vi "Create Map from Identifiers to Indexes.vi"(11 "RT hardware channel data":T2[](array[typedef]) {"labels settings for RT"."Label Timestamp Channel Data Reference" format="%.0x"; "labels settings for RT"."Word Initial Raw Value" format="%032.0f"; "labels settings for RT"."Label Disable/Trigger Channel Reference" format="%.0x"; "labels settings for RT"."parameter driver data"."Tx parameter refs" format="%.0x"; "labels settings for RT"."SDI" format="%02b"; "labels settings for RT"."label" format="%.0o"}) -> (3 "map from identifiers to indexes":T1)   [LabVIEW 2021, in "Ballard ARINC 429 Engine.lvlib" / "Custom Device.lvlib"]
uses:
  Custom Device.lvlib
  Shared/Map of Identifiers to Indexes.ctl
  Shared/Label.ctl
  <vilib>/NI/NI VeriStand Encoding and Decoding/Encoding.ctl
  <vilib>/NI/NI VeriStand Encoding and Decoding/Encoding and Decoding.lvlib
  Shared/Parameter Definition.ctl
  <vilib>/NI VeriStand/Custom Device API/Data Reference.ctl
  <vilib>/NI VeriStand/Custom Device API/Custom Device API.lvlib
  <vilib>/NI VeriStand/Custom Device API/Custom Device Item Ref.ctl
  Shared/RT Parameters.ctl
  Shared/Transfer Type.ctl
  Shared/RT Label Settings.ctl
  Shared/RT Hardware Channel Settings.ctl
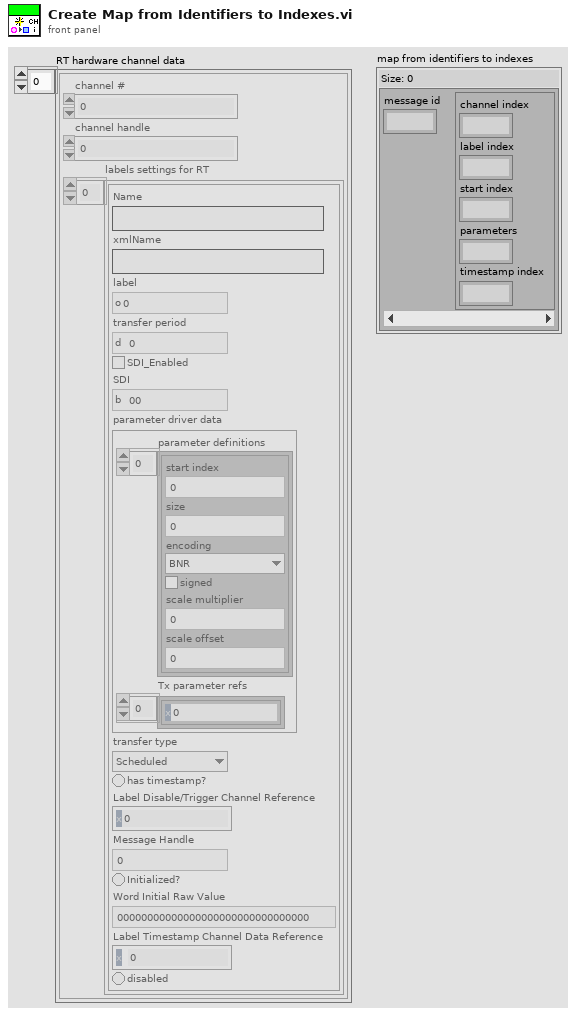
[diagram p1: front panel]
types:
  T1 = typedef "Map of Identifiers to Indexes.ctl" = map{u32, cluster{"channel index":i32, "label index":i32, "start index":i32, "parameters":i32, "timestamp index":i32}}
  T2 = typedef "RT Hardware Channel Settings.ctl" = cluster{"channel #":u16, "channel handle":u64, "labels settings for RT":T3[]}
  T3 = typedef "RT Label Settings.ctl" = cluster{"Name":string, "xmlName":string, "label":T4, "transfer period":u32, "SDI_Enabled":bool, "SDI":u8, "parameter driver data":T5, "transfer type":T9, "has timestamp?":bool, "Label Disable/Trigger Channel Reference":T8, "Message Handle":u64, "Initialized?":bool, "Word Initial Raw Value":u32, "Label Timestamp Channel Data Reference":T10, "disabled":bool}
  T4 = typedef "Label.ctl" = u8
  T5 = typedef "RT Parameters.ctl" = cluster{"parameter definitions":T6[], "Tx parameter refs":T8[]}
  T6 = typedef "Parameter Definition.ctl" = cluster{"start index":i32, "size":i32, "encoding":T7, "signed":bool, "scale multiplier":dbl, "scale offset":dbl}
  T7 = typedef "Encoding and Decoding.lvlib/Encoding.ctl" = enum16{"BNR", "BCD", "Discrete"}
  T8 = typedef "Custom Device API.lvlib/Custom Device Item Ref.ctl" = u64
  T9 = typedef "Transfer Type.ctl" = enum16{"Scheduled", "Acyclic", "Block", "Strobe"}
  T10 = typedef "Custom Device API.lvlib/Data Reference.ctl" = i32
  T11 = cluster{"channel index":i32, "label index":i32, "start index":i32, "parameters":i32, "timestamp index":i32}
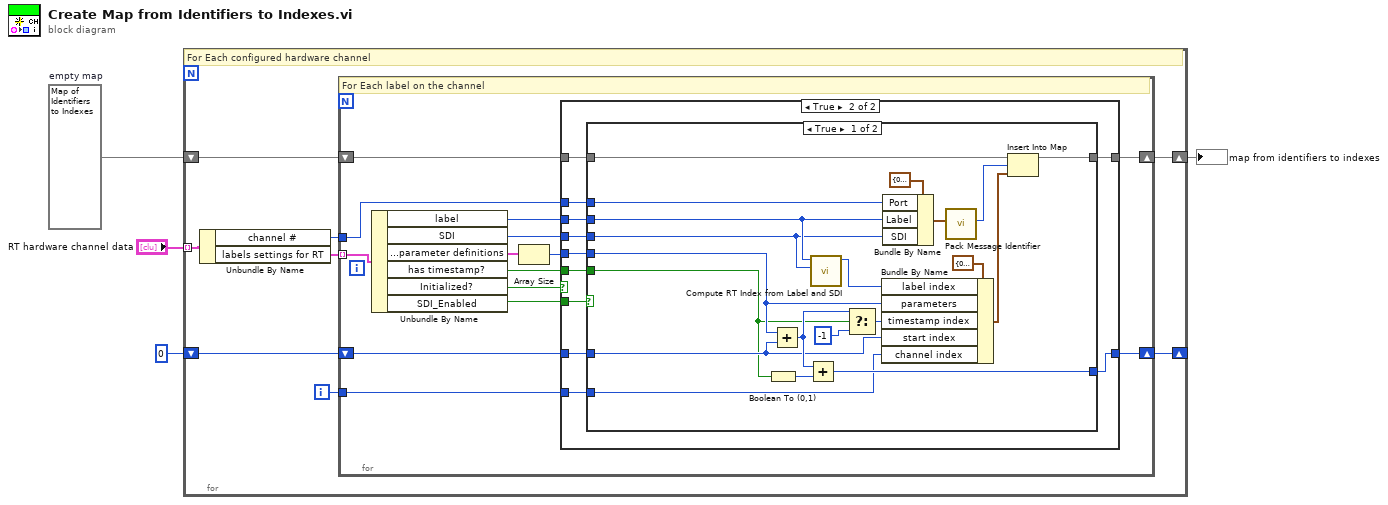
[diagram p0: block diagram]
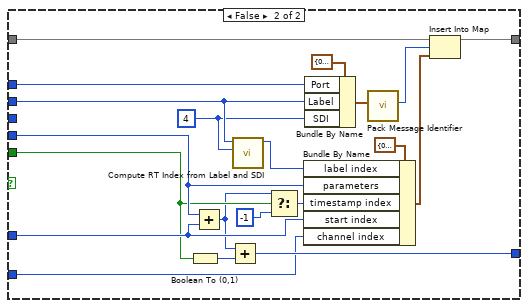
[diagram p3: hidden frame]
diagram:
  w3 = T1 {}  # empty map
  n1 = for {
    tunnel: "RT hardware channel data" -> [w12] mode=indexing
    shift-right: [w7] -> w2
    shift-left: w3 -> [w9]
    shift-right: [w6] -> _
    shift-left: 0 -> [w8]
    i -> [w5]
    # "For Each configured hardware channel"
    n2 = Unbundle By Name(w12) -> ("channel #"=w10:u16, "labels settings for RT"=w11:T3[])
    n3 = for {
      tunnel: w11 -> [w13] mode=indexing
      tunnel: w10 -> [w24]
      shift-right: [w18] -> w7
      shift-left: w9 -> [w21]
      shift-right: [w19] -> w6
      shift-left: w8 -> [w23]
      tunnel: w5 -> [w16]
      # "For Each label on the channel"
      n4 = Unbundle By Name(w13) -> ("label"=w25:T4, "SDI"=w20:u8, "parameter driver data.parameter definitions"=w26:T6[], "has timestamp?"=w15:bool, "Initialized?"=w17:bool, "SDI_Enabled"=w14:bool)
      n5 = Array Size(array=w26) -> (size(s)=w22:i32)
      n6 = case shown="True" w17 {
        tunnel: w25 -> [_ w35]
        tunnel: w24 -> [_ w38]
        tunnel: w23 -> [w27 w31]
        tunnel: w22 -> [_ w32]
        tunnel: w21 -> [w28 w39]
        tunnel: w20 -> [_ w34]
        tunnel: [w27 w37] -> w19
        tunnel: [w28 w36] -> w18
        tunnel: w16 -> [_ w33]
        tunnel: w15 -> [_ w30]
        tunnel: w14 -> [_ w29]
        frame False {
        }
        frame True {
          n7 = case shown="True" w29 {
            tunnel: w39 -> [w59 w79]
            tunnel: w38 -> [w58 w62]
            tunnel: [w56 w78] -> w37
            tunnel: [w55 w77] -> w36
            tunnel: w35 -> [w52 w61]
            tunnel: w34 -> [w51 _]
            tunnel: w33 -> [w49 w76]
            tunnel: w32 -> [w45 w75]
            tunnel: w31 -> [w43 w74]
            tunnel: w30 -> [w42 w73]
            frame True {
              n8 = Boolean To (0,1)(Boolean=w42) -> (0, 1=w48:i16)
              n9 = Add(x=w45, y=w43) -> (x+y=w46:i32)
              n10 = Add(x=w46, y=w48) -> (x+y=w56:i32)
              n11 = call "Compute RT Index from Label and SDI.vi"("SDI"=w51, "label"=w52) -> ("RT label index"=w50:i32)  [unwired: 9 in]
              n12 = Select(t=w46, s=w42, f=-1) -> (s? t:f=w47:i32)
              n13 = Bundle By Name(cluster=T11 {"channel index"=0, "label index"=0, "start index"=0, "parameters"=0, "timestamp index"=0} ("value"), "label index"=w50, "parameters"=w45, "timestamp index"=w47, "start index"=w43, "channel index"=w49) -> (w53:T11)
              n14 = Bundle By Name(cluster=cluster{"Port":u8, "Label":u8, "SDI":u8} {"Port"=0, "Label"=0, "SDI"=0} ("key"), "Port"=w58, "Label"=w52, "SDI"=w51) -> (w41:cluster{"Port":u8, "Label":u8, "SDI":u8})
              n15 = call "Pack Message Identifier.vi"("message identifiers"=w41) -> ("packed message identifier"=w40:u32)  [unwired: 10 in]
              n16 = Insert Into Map(map in=w59, key=w40, value=w53) -> (map out=w55:T1)  [unwired: 2 out]
            }
            frame False {
              w60 = u8 4 ("SDI")
              n17 = Boolean To (0,1)(Boolean=w73) -> (0, 1=w68:i16)
              n18 = Add(x=w75, y=w74) -> (x+y=w66:i32)
              n19 = Add(x=w66, y=w68) -> (x+y=w78:i32)
              n20 = call "Compute RT Index from Label and SDI.vi"("SDI"=w60, "label"=w61) -> ("RT label index"=w69:i32)  [unwired: 9 in]
              n21 = Select(t=w66, s=w73, f=-1) -> (s? t:f=w67:i32)
              n22 = Bundle By Name(cluster=T11 {"channel index"=0, "label index"=0, "start index"=0, "parameters"=0, "timestamp index"=0} ("value"), "label index"=w69, "parameters"=w75, "timestamp index"=w67, "start index"=w74, "channel index"=w76) -> (w70:T11)
              n23 = Bundle By Name(cluster=cluster{"Port":u8, "Label":u8, "SDI":u8} {"Port"=0, "Label"=0, "SDI"=0} ("key"), "Port"=w62, "Label"=w61, "SDI"=w60) -> (w64:cluster{"Port":u8, "Label":u8, "SDI":u8})
              n24 = call "Pack Message Identifier.vi"("message identifiers"=w64) -> ("packed message identifier"=w63:u32)  [unwired: 10 in]
              n25 = Insert Into Map(map in=w79, key=w63, value=w70) -> (map out=w77:T1)  [unwired: 2 out]
            }
          }
        }
      }
    }
  }
  "map from identifiers to indexes" <- w2
